vi "UpdateFreezedDropletImages.vi"(8 "error in (no error)":errorcluster, 9 "DropletNumber":u32, 10 "FreezeRelTime(sec)":u32, 11 "FreezedImageArray":cluster{"Image":u8[][]}[](array[cluster])) -> (0 "error out":errorcluster, 3 "OutputFreezedImagesRef":T1[](array[typedef]))   [LabVIEW 2013]
doc: "Use this template to build a VI to use as a subVI."
uses:
  <vilib>/vision/Image Controls.llb/IMAQ Image.ctl
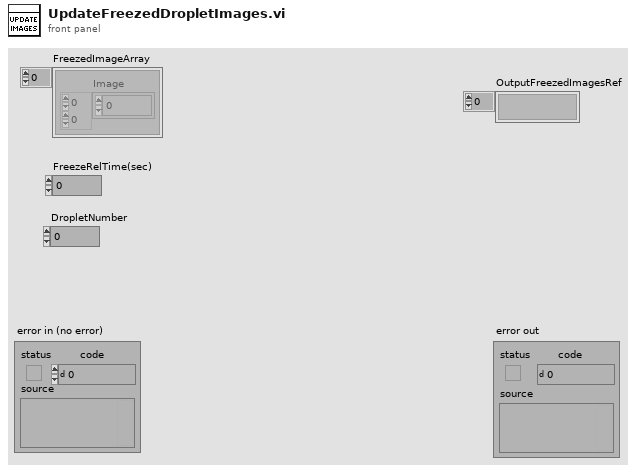
[diagram p1: front panel]
types:
  T1 = typedef "IMAQ Image.ctl" = refnum<image>
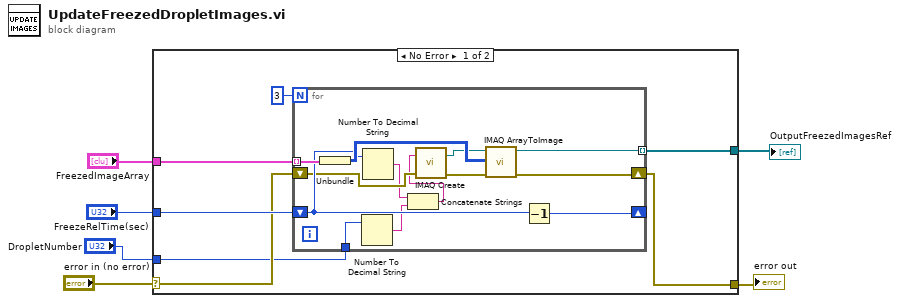
[diagram p0: block diagram]
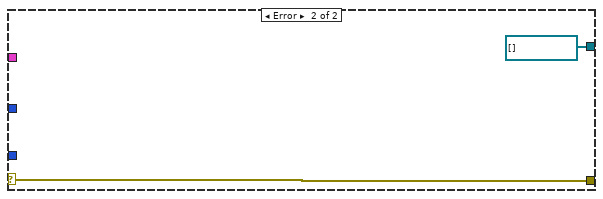
[diagram p2: hidden frame]
diagram:
  n1 = case shown="No Error" "error in (no error)" {
    selector: "error in (no error)" -> [w9 w28]
    tunnel: [w8 w28] -> w5
    tunnel: "FreezedImageArray" -> [w12 _]
    tunnel: "FreezeRelTime(sec)" -> [w11 _]
    tunnel: [w10 T1[] []] -> w2
    tunnel: "DropletNumber" -> [w7 _]
    frame No Error {
      n2 = for {
        N: 3 -> [_]
        tunnel: w12 -> [w26] mode=indexing
        shift-right: [w24] -> _
        shift-left: w11 -> [w23]
        tunnel: [w21] -> w10 mode=indexing
        shift-right: [w18] -> w8
        shift-left: w9 -> [w20]
        tunnel: w7 -> [w14]
        n3 = Unbundle(w26) -> ("Image"=w25:u8[][])
        n4 = Number To Decimal String(number=w14) -> (decimal integer string=w17:string)  [unwired: 1 in]
        n5 = Number To Decimal String(number=w23) -> (decimal integer string=w16:string)  [unwired: 1 in]
        n6 = Concatenate Strings(w16, w17) -> (w15:string)
        n7 = call "IMAQ Create"("Image Name"=w15, "error in (no error)"=w20) -> ("New Image"=w22:T1, "error out"=w19:errorcluster)  [unwired: 2 in, 1 out]
        n8 = call "IMAQ ArrayToImage"("error in (no error)"=w19, "Image Pixels (U8)"=w25, "Image"=w22) -> ("error out"=w18:errorcluster, "Image Out"=w21:T1)  [unwired: 7 in]
        n9 = Decrement(x=w23) -> (x-1=w24:u32)
      }
    }
    frame Error {
    }
  }
  "error out" <- w5
  "OutputFreezedImagesRef" <- w2
